vi "CalculateHighpassPkPk.vi"(8 "error in (no error)":errorcluster, 10 "waveform in":waveform(sgl), 11 "Feature":T1) -> (0 "error out":errorcluster, 1 "valid":bool, 2 "value":dbl, 3 "Feature out":T1)   [LabVIEW 2017, in "AnalysisHelper.lvlib"]
uses:
  <vilib>/addons/InsightCM/Utilities/Analysis/Shared/AnalysisHelper.lvlib
  <vilib>/addons/InsightCM/Utilities/Analysis/Shared/controls/Feature.ctl
  <vilib>/addons/InsightCM/Utilities/Analysis/Shared/controls/AmplitudeScale.ctl
  <vilib>/addons/InsightCM/Utilities/Analysis/Vibration/controls/HighPassFilterState.ctl
  <vilib>/addons/InsightCM/Utilities/Analysis/Vibration/VibrationAnalysisFunctions.lvlib
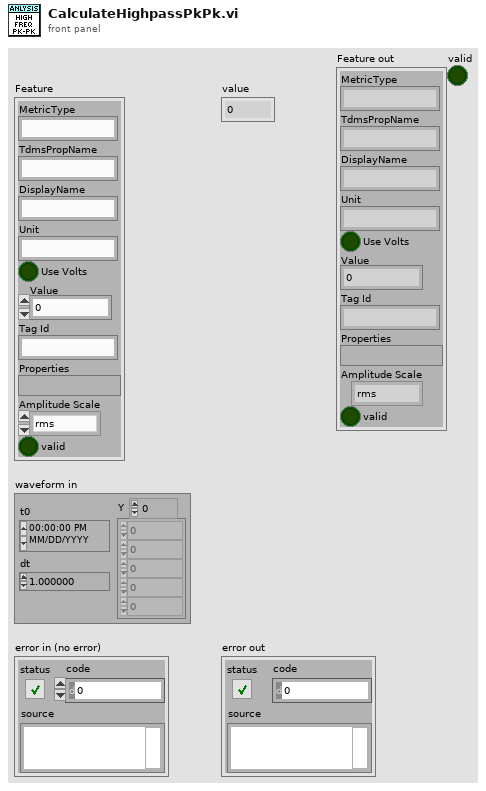
[diagram p1: front panel]
types:
  T1 = typedef "AnalysisHelper.lvlib/Feature.ctl" = cluster{"MetricType":string, "TdmsPropName":string, "DisplayName":string, "Unit":string, "Use Volts":bool, "Value":dbl, "Tag Id":string, "Properties":variant, "Amplitude Scale":T2, "valid":bool}
  T2 = typedef "AnalysisHelper.lvlib/AmplitudeScale.ctl" = enum16{"rms", "peak", "pk-pk"}
  T3 = typedef "VibrationAnalysisFunctions.lvlib/HighPassFilterState.ctl" = cluster{"designed":bool, "IIR Filter Cluster":cluster{"filter structure":enum32{"IIR 2nd Order", "IIR 4th Order"}, "Reverse Coefficients":dbl[], "Forward Coefficients":dbl[]}, "Filter State":dbl[]}
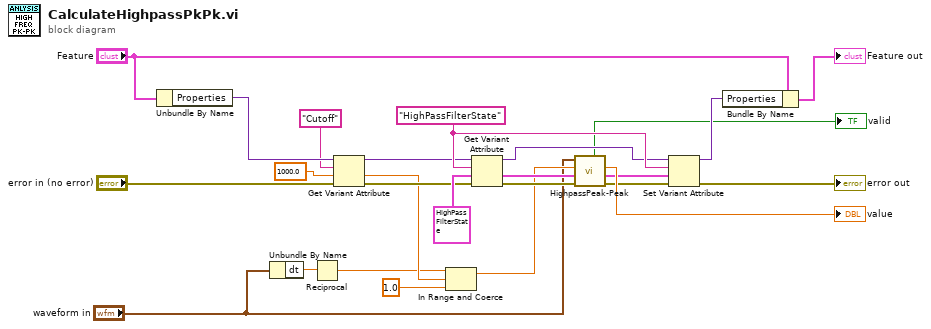
[diagram p0: block diagram]
diagram:
  w17 = "HighPassFilterState" ("name")
  n1 = Unbundle By Name("Feature") -> ("Properties"=w11:variant)
  n2 = Unbundle By Name("waveform in") -> ("dt"=w3:dbl)
  n3 = Reciprocal(x=w3) -> (1/x=w1:dbl)
  n4 = Get Variant Attribute(Variant=w11, name="Cutoff", default value (empty Variant)=1000.0 ("highpass cutoff"), error in="error in (no error)") -> (duplicate Variant=w10:variant, value=w6:dbl, error out=w12:errorcluster)  [unwired: 1 out]
  n5 = In Range and Coerce(upper limit=w1, x=w6, lower limit=1.0 ("upper limit")) -> (coerced(x)=w5:dbl)  [unwired: 1 out]
  n6 = Get Variant Attribute(Variant=w10, name=w17, default value (empty Variant)=T3 {"designed"=FALSE, "IIR Filter Cluster"={"filter structure"=enum."IIR 2nd Order", "Reverse Coefficients"=[], "Forward Coefficients"=[]}, "Filter State"=[]} ("Highpass Filter State"), error in=w12) -> (duplicate Variant=w15:variant, value=w22:T3, error out=w24:errorcluster)  [unwired: 1 out]
  n7 = call <vilib>:"HighpassPeak-Peak.vi"("error in (no error)"=w24, "Highpass Filter State"=w22, "highpass cutoff"=w5, "input signal"="waveform in") -> ("error out"=w19:errorcluster, "Highpass Filter State out"=w16:T3, "pk-pk"=→"value":dbl, "valid"=→"valid":bool)  [unwired: 4 in]
  n8 = Set Variant Attribute(Variant=w15, name=w17, value=w16, error in=w19) -> (Variant out=w14:variant, error out=→"error out":errorcluster)  [unwired: 1 out]
  n9 = Bundle By Name(cluster="Feature", "Properties"=w14) -> (→"Feature out":T1)
